vi "FT10_Triverse Tester.vi"() -> ()   [LabVIEW 2024]
uses:
  <vilib>/rvi/interface/nirviOpenFPGA/nirviOpenFPGA.xnode
  <vilib>/rvi/interface/nirviReadWriteControl/nirviReadWriteControl.xnode
  <vilib>/rvi/interface/nirviCloseFPGA/nirviCloseFPGA.xnode
  FPGA Bitfiles/11_12_2024_FT10_FPGA_7854R_Main_Rev3 BitFile.lvbitx
  <vilib>/FPGAPlugInAG/PXI-7854R/niLvFpga_Open_PXI-7854R.vi
  <vilib>/rvi/interface/common/dynamic/niFpgaDynamicAddResources.vi
  <vilib>/FPGAPlugInAG/Dynamic/niLvFpga_Close_Dynamic.vi
  NiFpgaLv.dll
  <vilib>/Utility/error.llb/Error Cluster From Error Code.vi
  <vilib>/rvi/interface/Simulation/niFpgaSimulationCallBeginRW.vi
  <vilib>/rvi/errors/niLvFpgaAdjustHostInterfaceError.vi
panel:
  in  "Triverse Mode":T1(ring)
  out "error out":errorcluster
  in  "error in":errorcluster
  in  "stop":bool
  in  "uSec On":u16
  in  "uSec Off":u16
  in  "75kHz":bool
  in  "Conn2/DIO_0_7 In":bool[](array[boolean])=[FALSE, FALSE, FALSE, FALSE, FALSE, FALSE, FALSE, FALSE]
  in  "Conn2/DIO_8_15 In":bool[](array[boolean])=[FALSE, FALSE, FALSE, FALSE, FALSE, FALSE, FALSE, FALSE]
  out "Conn2/DIO_0_7 Out":bool[](array[boolean])
  out "Conn2/DIO_8_15 Out":bool[](array[boolean])
  out "error out 2":errorcluster
  out "Conn2/DIO_16_23 Out":bool[](array[boolean])
  in  "Conn2/DIO_16_23 In":bool[](array[boolean])=[FALSE, FALSE, FALSE, FALSE, FALSE, FALSE, FALSE, FALSE]
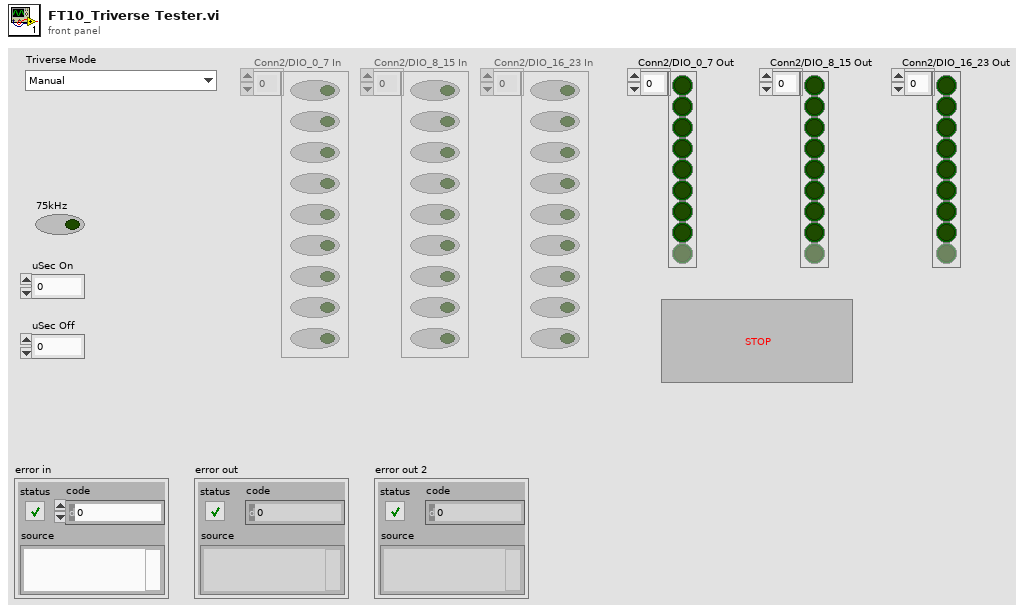
[diagram p1: front panel]
types:
  T1 = enum16{"Manual", "Enter Triverse Mode", "Set Potentiometer R32", "Set Potentiometer R31", "Intensity A P5", "Intensity A P4", "Intensity A P3", "Intensity A P2", "Intensity A P1", "Intensity B P5", "Intensity B P4", "Intensity B P3", "Intensity B P2", "Intensity B P1", "Mode A S3 Coag", "Mode A S2 Valleylab", "Mode A S1 Cut", "Mode B S3 Coag", "Mode B S2 Valleylab", "Mode B S1 Cut"}
  T2 = enum8{"Enabled", "Disabled", "Disabled and Grayed Out"}
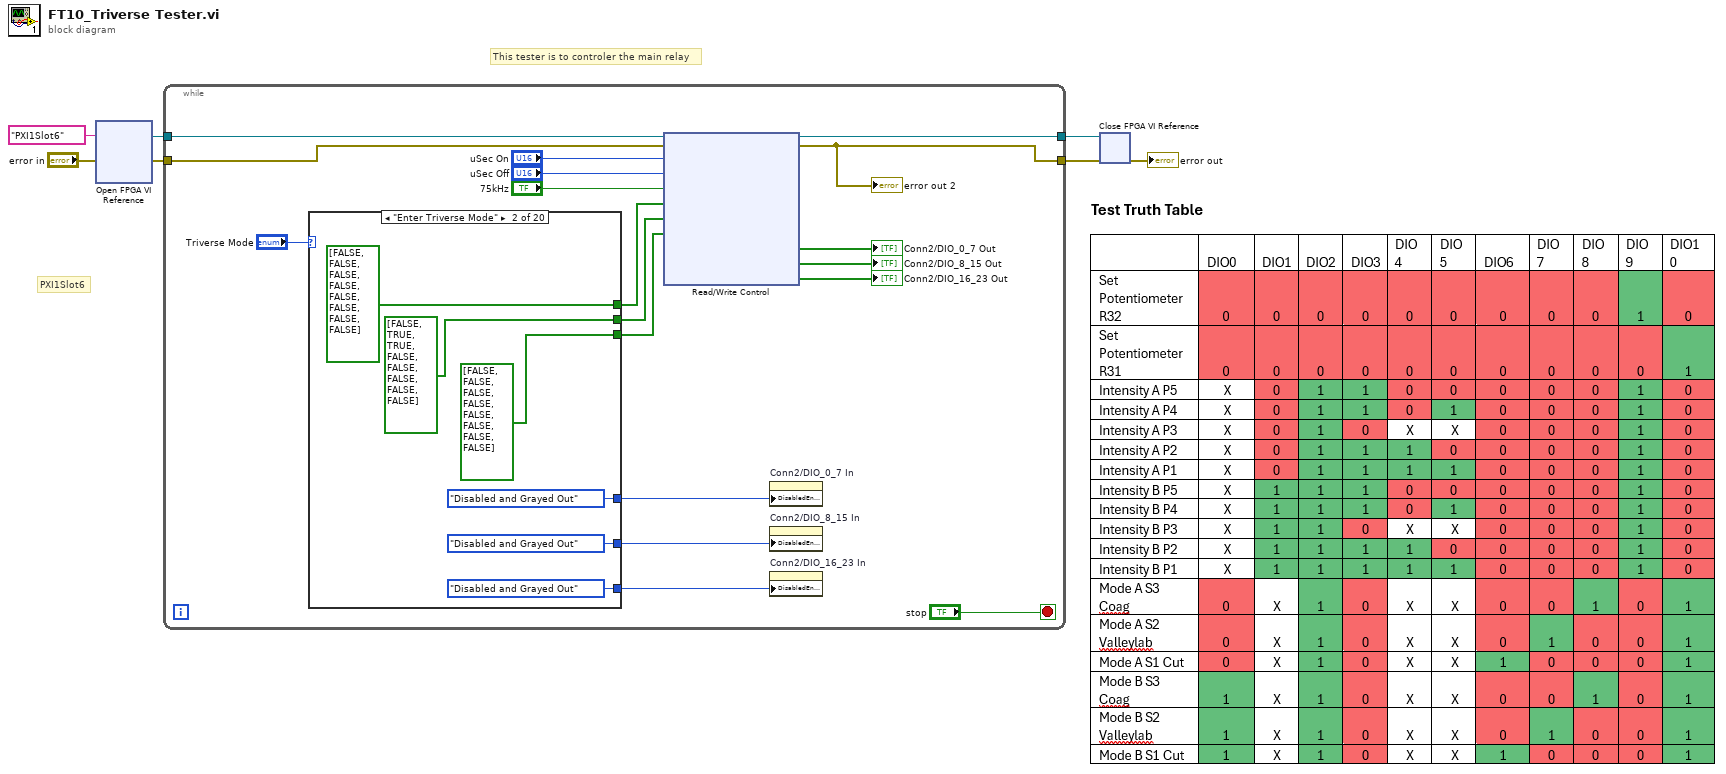
[diagram p0: block diagram]
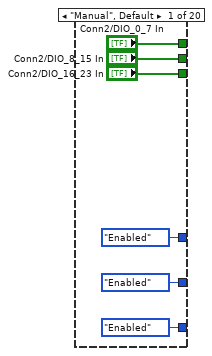
[diagram p2: hidden frame]
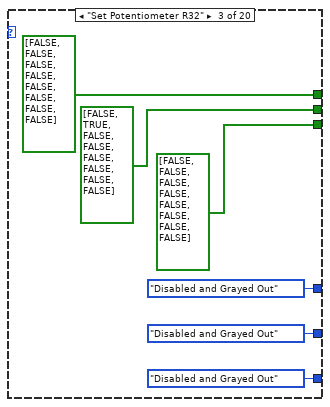
[diagram p3: hidden frame]
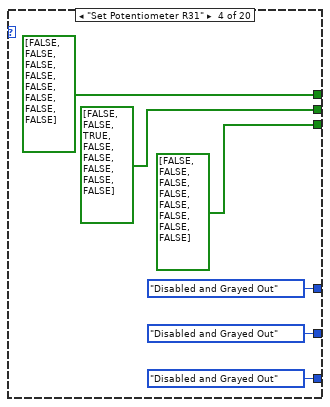
[diagram p4: hidden frame]
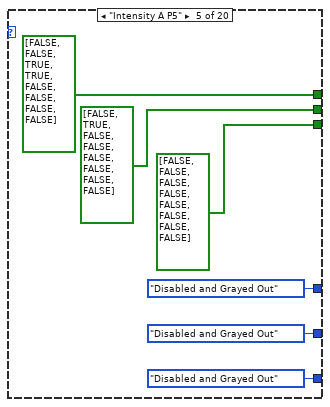
[diagram p5: hidden frame]
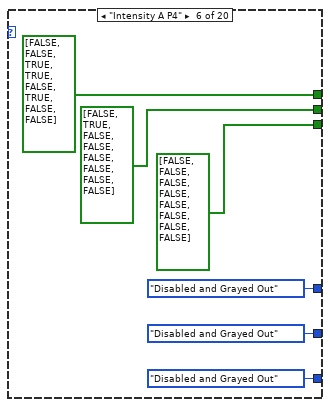
[diagram p6: hidden frame]
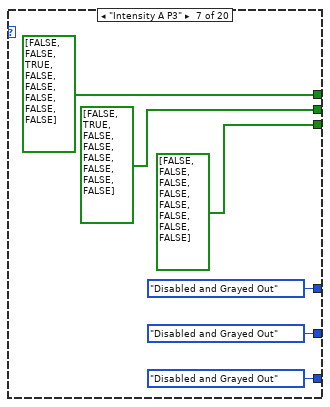
[diagram p7: hidden frame]
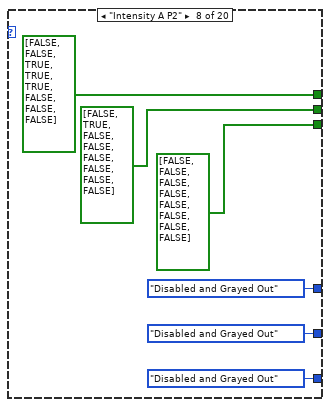
[diagram p8: hidden frame]
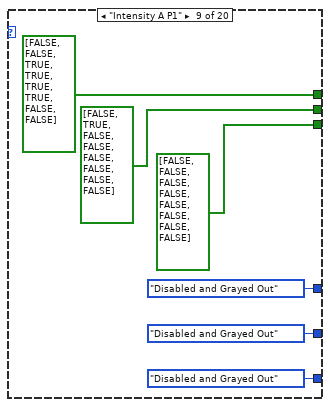
[diagram p9: hidden frame]
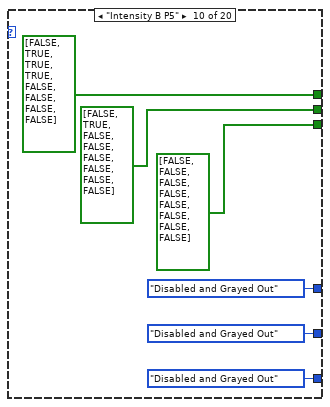
[diagram p10: hidden frame]
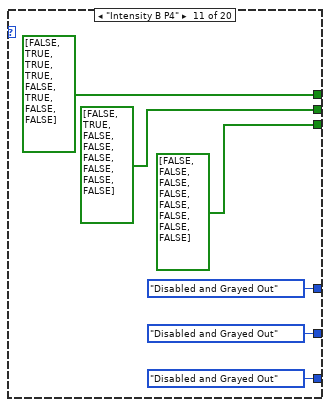
[diagram p11: hidden frame]
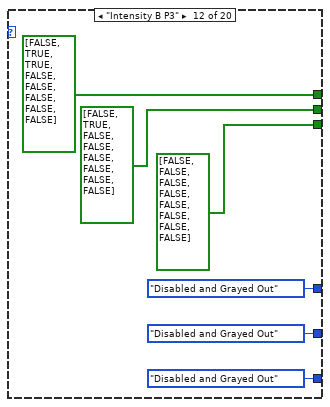
[diagram p12: hidden frame]
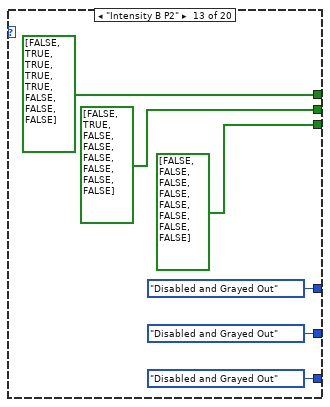
[diagram p13: hidden frame]
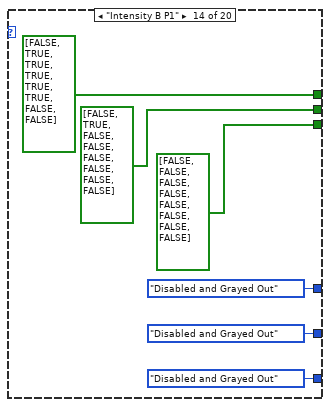
[diagram p14: hidden frame]
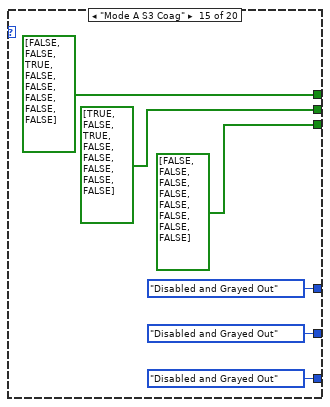
[diagram p15: hidden frame]
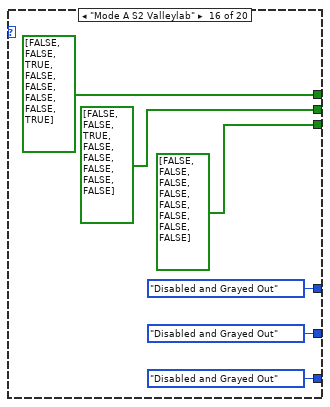
[diagram p16: hidden frame]
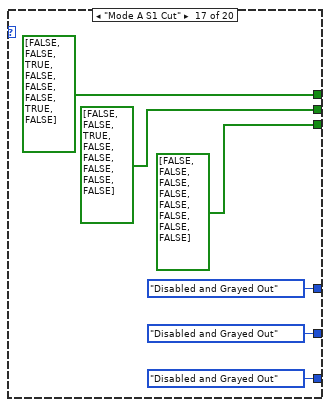
[diagram p17: hidden frame]
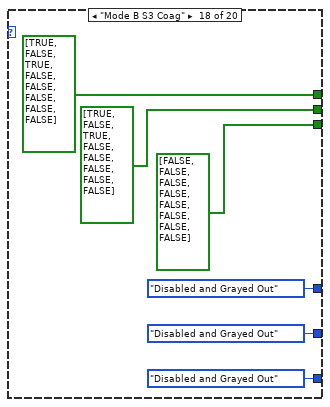
[diagram p18: hidden frame]
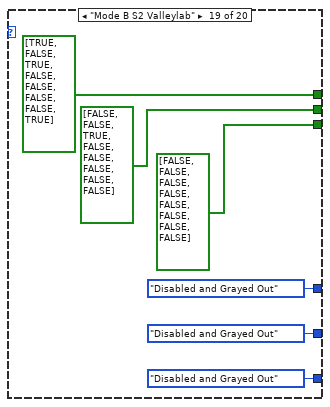
[diagram p19: hidden frame]
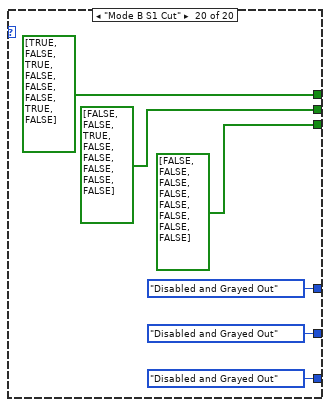
[diagram p20: hidden frame]
diagram:
  # "PXI1Slot6"
  # "This tester is to controler the main relay"
  n1 = xnode "Open FPGA VI Reference"("error in"="error in", "resource name"=tag "PXI1Slot6") -> ("FPGA VI Reference Out"=w1:refnum<k20>, "error out"=w2:errorcluster)
  n2 = while {
    tunnel: w1 -> [w25]
    tunnel: [w24] -> w7
    tunnel: w2 -> [w23]
    tunnel: [w22] -> w6
    stop <- "stop" stop-if-true
    n3 = case shown="\"Enter Triverse Mode\"" "Triverse Mode" {
      tunnel: ["Conn2/DIO_0_7 In" bool[] [FALSE, FALSE, FALSE, FALSE, FALSE, FALSE, FALSE, FALSE] ("Conn2/DIO_0_7 In") bool[] [FALSE, FALSE, FALSE, FALSE, FALSE, FALSE, FALSE, FALSE] ("Conn2/DIO_0_7 In") bool[] [FALSE, FALSE, FALSE, FALSE, FALSE, FALSE, FALSE, FALSE] ("Conn2/DIO_0_7 In") bool[] [FALSE, FALSE, TRUE, TRUE, FALSE, FALSE, FALSE, FALSE] ("Conn2/DIO_0_7 In") bool[] [FALSE, FALSE, TRUE, TRUE, FALSE, TRUE, FALSE, FALSE] ("Conn2/DIO_0_7 In") bool[] [FALSE, FALSE, TRUE, FALSE, FALSE, FALSE, FALSE, FALSE] ("Conn2/DIO_0_7 In") bool[] [FALSE, FALSE, TRUE, TRUE, TRUE, FALSE, FALSE, FALSE] ("Conn2/DIO_0_7 In") bool[] [FALSE, FALSE, TRUE, TRUE, TRUE, TRUE, FALSE, FALSE] ("Conn2/DIO_0_7 In") bool[] [FALSE, TRUE, TRUE, TRUE, FALSE, FALSE, FALSE, FALSE] ("Conn2/DIO_0_7 In") bool[] [FALSE, TRUE, TRUE, TRUE, FALSE, TRUE, FALSE, FALSE] ("Conn2/DIO_0_7 In") bool[] [FALSE, TRUE, TRUE, FALSE, FALSE, FALSE, FALSE, FALSE] ("Conn2/DIO_0_7 In") bool[] [FALSE, TRUE, TRUE, TRUE, TRUE, FALSE, FALSE, FALSE] ("Conn2/DIO_0_7 In") bool[] [FALSE, TRUE, TRUE, TRUE, TRUE, TRUE, FALSE, FALSE] ("Conn2/DIO_0_7 In") bool[] [FALSE, FALSE, TRUE, FALSE, FALSE, FALSE, FALSE, FALSE] ("Conn2/DIO_0_7 In") bool[] [FALSE, FALSE, TRUE, FALSE, FALSE, FALSE, FALSE, TRUE] ("Conn2/DIO_0_7 In") bool[] [FALSE, FALSE, TRUE, FALSE, FALSE, FALSE, TRUE, FALSE] ("Conn2/DIO_0_7 In") bool[] [TRUE, FALSE, TRUE, FALSE, FALSE, FALSE, FALSE, FALSE] ("Conn2/DIO_0_7 In") bool[] [TRUE, FALSE, TRUE, FALSE, FALSE, FALSE, FALSE, TRUE] ("Conn2/DIO_0_7 In") bool[] [TRUE, FALSE, TRUE, FALSE, FALSE, FALSE, TRUE, FALSE] ("Conn2/DIO_0_7 In")] -> w17
      tunnel: ["Conn2/DIO_8_15 In" bool[] [FALSE, TRUE, TRUE, FALSE, FALSE, FALSE, FALSE, FALSE] ("Conn2/DIO_0_7 In") bool[] [FALSE, TRUE, FALSE, FALSE, FALSE, FALSE, FALSE, FALSE] ("Conn2/DIO_0_7 In") bool[] [FALSE, FALSE, TRUE, FALSE, FALSE, FALSE, FALSE, FALSE] ("Conn2/DIO_0_7 In") bool[] [FALSE, TRUE, FALSE, FALSE, FALSE, FALSE, FALSE, FALSE] ("Conn2/DIO_0_7 In") bool[] [FALSE, TRUE, FALSE, FALSE, FALSE, FALSE, FALSE, FALSE] ("Conn2/DIO_0_7 In") bool[] [FALSE, TRUE, FALSE, FALSE, FALSE, FALSE, FALSE, FALSE] ("Conn2/DIO_0_7 In") bool[] [FALSE, TRUE, FALSE, FALSE, FALSE, FALSE, FALSE, FALSE] ("Conn2/DIO_0_7 In") bool[] [FALSE, TRUE, FALSE, FALSE, FALSE, FALSE, FALSE, FALSE] ("Conn2/DIO_0_7 In") bool[] [FALSE, TRUE, FALSE, FALSE, FALSE, FALSE, FALSE, FALSE] ("Conn2/DIO_0_7 In") bool[] [FALSE, TRUE, FALSE, FALSE, FALSE, FALSE, FALSE, FALSE] ("Conn2/DIO_0_7 In") bool[] [FALSE, TRUE, FALSE, FALSE, FALSE, FALSE, FALSE, FALSE] ("Conn2/DIO_0_7 In") bool[] [FALSE, TRUE, FALSE, FALSE, FALSE, FALSE, FALSE, FALSE] ("Conn2/DIO_0_7 In") bool[] [FALSE, TRUE, FALSE, FALSE, FALSE, FALSE, FALSE, FALSE] ("Conn2/DIO_0_7 In") bool[] [TRUE, FALSE, TRUE, FALSE, FALSE, FALSE, FALSE, FALSE] ("Conn2/DIO_0_7 In") bool[] [FALSE, FALSE, TRUE, FALSE, FALSE, FALSE, FALSE, FALSE] ("Conn2/DIO_0_7 In") bool[] [FALSE, FALSE, TRUE, FALSE, FALSE, FALSE, FALSE, FALSE] ("Conn2/DIO_0_7 In") bool[] [TRUE, FALSE, TRUE, FALSE, FALSE, FALSE, FALSE, FALSE] ("Conn2/DIO_0_7 In") bool[] [FALSE, FALSE, TRUE, FALSE, FALSE, FALSE, FALSE, FALSE] ("Conn2/DIO_0_7 In") bool[] [FALSE, FALSE, TRUE, FALSE, FALSE, FALSE, FALSE, FALSE] ("Conn2/DIO_0_7 In")] -> w16
      tunnel: ["Conn2/DIO_16_23 In" bool[] [FALSE, FALSE, FALSE, FALSE, FALSE, FALSE, FALSE, FALSE] ("Conn2/DIO_0_7 In") bool[] [FALSE, FALSE, FALSE, FALSE, FALSE, FALSE, FALSE, FALSE] ("Conn2/DIO_0_7 In") bool[] [FALSE, FALSE, FALSE, FALSE, FALSE, FALSE, FALSE, FALSE] ("Conn2/DIO_0_7 In") bool[] [FALSE, FALSE, FALSE, FALSE, FALSE, FALSE, FALSE, FALSE] ("Conn2/DIO_0_7 In") bool[] [FALSE, FALSE, FALSE, FALSE, FALSE, FALSE, FALSE, FALSE] ("Conn2/DIO_0_7 In") bool[] [FALSE, FALSE, FALSE, FALSE, FALSE, FALSE, FALSE, FALSE] ("Conn2/DIO_0_7 In") bool[] [FALSE, FALSE, FALSE, FALSE, FALSE, FALSE, FALSE, FALSE] ("Conn2/DIO_0_7 In") bool[] [FALSE, FALSE, FALSE, FALSE, FALSE, FALSE, FALSE, FALSE] ("Conn2/DIO_0_7 In") bool[] [FALSE, FALSE, FALSE, FALSE, FALSE, FALSE, FALSE, FALSE] ("Conn2/DIO_0_7 In") bool[] [FALSE, FALSE, FALSE, FALSE, FALSE, FALSE, FALSE, FALSE] ("Conn2/DIO_0_7 In") bool[] [FALSE, FALSE, FALSE, FALSE, FALSE, FALSE, FALSE, FALSE] ("Conn2/DIO_0_7 In") bool[] [FALSE, FALSE, FALSE, FALSE, FALSE, FALSE, FALSE, FALSE] ("Conn2/DIO_0_7 In") bool[] [FALSE, FALSE, FALSE, FALSE, FALSE, FALSE, FALSE, FALSE] ("Conn2/DIO_0_7 In") bool[] [FALSE, FALSE, FALSE, FALSE, FALSE, FALSE, FALSE, FALSE] ("Conn2/DIO_0_7 In") bool[] [FALSE, FALSE, FALSE, FALSE, FALSE, FALSE, FALSE, FALSE] ("Conn2/DIO_0_7 In") bool[] [FALSE, FALSE, FALSE, FALSE, FALSE, FALSE, FALSE, FALSE] ("Conn2/DIO_0_7 In") bool[] [FALSE, FALSE, FALSE, FALSE, FALSE, FALSE, FALSE, FALSE] ("Conn2/DIO_0_7 In") bool[] [FALSE, FALSE, FALSE, FALSE, FALSE, FALSE, FALSE, FALSE] ("Conn2/DIO_0_7 In") bool[] [FALSE, FALSE, FALSE, FALSE, FALSE, FALSE, FALSE, FALSE] ("Conn2/DIO_0_7 In")] -> w13
      tunnel: [T2."Enabled" ("Disabled") T2."Disabled and Grayed Out" ("Disabled") T2."Disabled and Grayed Out" ("Disabled") T2."Disabled and Grayed Out" ("Disabled") T2."Disabled and Grayed Out" ("Disabled") T2."Disabled and Grayed Out" ("Disabled") T2."Disabled and Grayed Out" ("Disabled") T2."Disabled and Grayed Out" ("Disabled") T2."Disabled and Grayed Out" ("Disabled") T2."Disabled and Grayed Out" ("Disabled") T2."Disabled and Grayed Out" ("Disabled") T2."Disabled and Grayed Out" ("Disabled") T2."Disabled and Grayed Out" ("Disabled") T2."Disabled and Grayed Out" ("Disabled") T2."Disabled and Grayed Out" ("Disabled") T2."Disabled and Grayed Out" ("Disabled") T2."Disabled and Grayed Out" ("Disabled") T2."Disabled and Grayed Out" ("Disabled") T2."Disabled and Grayed Out" ("Disabled") T2."Disabled and Grayed Out" ("Disabled")] -> w10
      tunnel: [T2."Enabled" ("Disabled") T2."Disabled and Grayed Out" ("Disabled") T2."Disabled and Grayed Out" ("Disabled") T2."Disabled and Grayed Out" ("Disabled") T2."Disabled and Grayed Out" ("Disabled") T2."Disabled and Grayed Out" ("Disabled") T2."Disabled and Grayed Out" ("Disabled") T2."Disabled and Grayed Out" ("Disabled") T2."Disabled and Grayed Out" ("Disabled") T2."Disabled and Grayed Out" ("Disabled") T2."Disabled and Grayed Out" ("Disabled") T2."Disabled and Grayed Out" ("Disabled") T2."Disabled and Grayed Out" ("Disabled") T2."Disabled and Grayed Out" ("Disabled") T2."Disabled and Grayed Out" ("Disabled") T2."Disabled and Grayed Out" ("Disabled") T2."Disabled and Grayed Out" ("Disabled") T2."Disabled and Grayed Out" ("Disabled") T2."Disabled and Grayed Out" ("Disabled") T2."Disabled and Grayed Out" ("Disabled")] -> w9
      tunnel: [T2."Enabled" ("Disabled") T2."Disabled and Grayed Out" ("Disabled") T2."Disabled and Grayed Out" ("Disabled") T2."Disabled and Grayed Out" ("Disabled") T2."Disabled and Grayed Out" ("Disabled") T2."Disabled and Grayed Out" ("Disabled") T2."Disabled and Grayed Out" ("Disabled") T2."Disabled and Grayed Out" ("Disabled") T2."Disabled and Grayed Out" ("Disabled") T2."Disabled and Grayed Out" ("Disabled") T2."Disabled and Grayed Out" ("Disabled") T2."Disabled and Grayed Out" ("Disabled") T2."Disabled and Grayed Out" ("Disabled") T2."Disabled and Grayed Out" ("Disabled") T2."Disabled and Grayed Out" ("Disabled") T2."Disabled and Grayed Out" ("Disabled") T2."Disabled and Grayed Out" ("Disabled") T2."Disabled and Grayed Out" ("Disabled") T2."Disabled and Grayed Out" ("Disabled") T2."Disabled and Grayed Out" ("Disabled")] -> w8
      frame "Manual", Default {
      }
      frame "Enter Triverse Mode" {
      }
      frame "Set Potentiometer R32" {
      }
      frame "Set Potentiometer R31" {
      }
      frame "Intensity A P5" {
      }
      frame "Intensity A P4" {
      }
      frame "Intensity A P3" {
      }
      frame "Intensity A P2" {
      }
      frame "Intensity A P1" {
      }
      frame "Intensity B P5" {
      }
      frame "Intensity B P4" {
      }
      frame "Intensity B P3" {
      }
      frame "Intensity B P2" {
      }
      frame "Intensity B P1" {
      }
      frame "Mode A S3 Coag" {
      }
      frame "Mode A S2 Valleylab" {
      }
      frame "Mode A S1 Cut" {
      }
      frame "Mode B S3 Coag" {
      }
      frame "Mode B S2 Valleylab" {
      }
      frame "Mode B S1 Cut" {
      }
    }
    n4 = xnode "Read/Write Control"("FPGA VI Reference In"=w25, "error in"=w23, "Conn1 - uSec On"="uSec On", "Conn1 - uSec Off"="uSec Off", "Conn1 - 75kHz"="75kHz", "Conn1/DIO_0_7 In"=w17, "Conn1/DIO_8_15 In"=w16, "Conn1/DIO_16_23 In"=w13) -> ("FPGA VI Reference Out"=w24:refnum<k20>, "error out"=w22:errorcluster, "Conn1/DIO_0_7 Out"=→"Conn2/DIO_0_7 Out":bool[], "Conn1/DIO_8_15 Out"=→"Conn2/DIO_8_15 Out":bool[], "Conn1/DIO_16_23 Out"=→"Conn2/DIO_16_23 Out":bool[])
    "error out 2" <- w22
    n5 = property on="Conn2/DIO_0_7 In" class="Arr (strict)"("DisabledEnum"=w10) -> ()  [unwired: 2 in, 2 out]
    n6 = property on="Conn2/DIO_8_15 In" class="Arr (strict)"("DisabledEnum"=w9) -> ()  [unwired: 2 in, 2 out]
    n7 = property on="Conn2/DIO_16_23 In" class="Arr (strict)"("DisabledEnum"=w8) -> ()  [unwired: 2 in, 2 out]
  }
  n8 = xnode "Close FPGA VI Reference"("FPGA VI Reference In"=w7, "error in"=w6) -> ("error out"=→"error out":errorcluster)
